vi "Get Settings.vi"(8 "error in (no error)":errorcluster, 11 "Keithley 622x2182 Driver in":refnum<class "Keithley 622x2182 Driver.lvclass">) -> (0 "error out":errorcluster, 2 "Settings":string[](array[string]), 3 "Keithley 622x2182 Driver out":refnum<class "Keithley 622x2182 Driver.lvclass">)   [LabVIEW 2021, in "Keithley 622x2182 Driver.lvclass"]
uses:
  Keithley 622x2182 Driver.lvclass
  Keithley 622x2182 Driver.lvclass/Keithley 622x2182 Driver.ctl
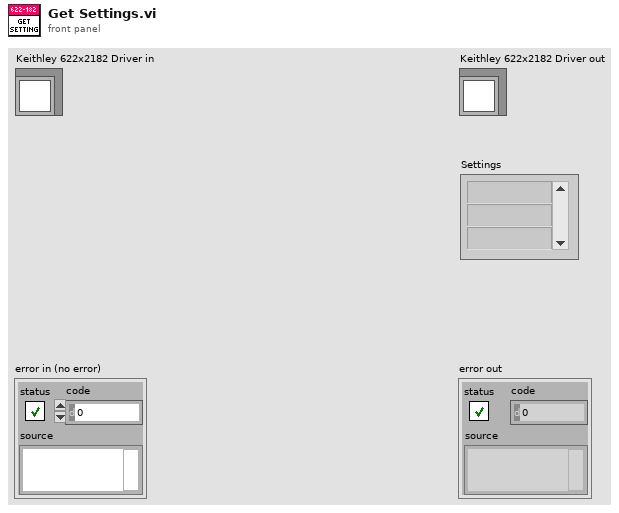
[diagram p1: front panel]
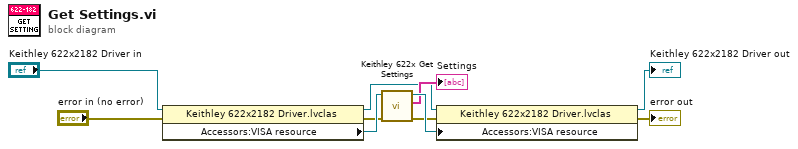
[diagram p0: block diagram]
diagram:
  n1 = property class="Keithley 622x2182 Driver.lvclas"(reference="Keithley 622x2182 Driver in", error in="error in (no error)") -> (reference out=w3:refnum<class "Keithley 622x2182 Driver.lvclass">, error out=w2:errorcluster, "Accessors:VISA resource"=w6:refnum<visa-resource-name>)
  n2 = call "Keithley 622x Get Settings.vi"("error in"=w2, "VISA resource name"=w6) -> ("error out"=w1:errorcluster, "Settings"=→"Settings":string[], "VISA resource name out"=w5:refnum<visa-resource-name>)  [unwired: 6 in, 1 out]
  n3 = property class="Keithley 622x2182 Driver.lvclas"(reference=w3, error in=w1, "Accessors:VISA resource"=w5) -> (reference out=→"Keithley 622x2182 Driver out":refnum<class "Keithley 622x2182 Driver.lvclass">, error out=→"error out":errorcluster)
